vi "Analiza położeń robotów.vi"(0 "Zapis danych z przejazdu":T3={"Łazik"=path "C:/Users/User/Desktop/Łazik/Zapis zebranych danych/Łazik.txt", "Quadron"=path "C:/Users/User/Desktop/Łazik/Zapis zebranych danych/Łazik.txt", "Dron 1"=path "C:/Users/User/Desktop/Łazik/Zapis zebranych danych/Łazik.txt", "Dron 2"=path "C:/Users/User/Desktop/Łazik/Zapis zebranych danych/Łazik.txt", "Sparus"=path "C:/Users/User/Desktop/Łazik/Zapis zebranych danych/Łazik.txt"}, 1 "Azymut łazika\n pocz/nowy":dbl caption="Azymut robota pocz/nowy" min=0.0 max=360.0, 5 "Parametry odwzorowania\n Ziemi (WGS84)":T8={"a"=6378137.0, "b"=6356752.3142} {"b" format="%#.6g"; "a" format="%#.6g"}, 7 "Ustawienia początkowe":T5, 9 "Poł. bazy.":T7={"UTM"={"E [m]"=276177.7293177693, "N [m]"=1172675.379150019, "Strefa"="38P"}, "Piksele"={"X"=991, "Y"=338}} {"UTM"."N [m]" format="%#_10g"}, 11 "Wybór robota":T4 items=["Łazik", "Quadron", "Dron 1", "Dron 2"], 12 "Reset":T1) -> (4 "Azymut":dbl(knob) scale=0.0..360.0, 6 "Odległość robota od bazy  [m]":cluster{"X [m]":dbl, "Y [m]":dbl}, 10 "Lokalizacja robotów":T6, 15 "Odczyt GPS - Łazik 2":T2 caption="Położenie wybranego robota" {"Szerokośc geograficzna \n- GPS" format="%_9f"; "Długość geograficzna \n- GPS" format="%_9f"; "Położenie \nrobota  UTM"."E [m]" format="%#_10g"; "Położenie \nrobota  UTM"."N [m]" format="%#_12g"})   [LabVIEW 2015, in "Biblioteka moduł map v3.lvlib" / "Pomocnicze.lvlib"]
uses:
  Pomocnicze.lvlib
  Kontrolki/Parametry odwzorowania Ziemi.ctl
  Zmienne/Lokalizacja GPS/longitude Quadron.vi
  Zmienne/Lokalizacja GPS/latitude Quadron.vi
  Zmienne/Lokalizacja GPS/Longitude dron 1.vi
  Zmienne/Lokalizacja GPS/Latitude dron 1.vi
  Zmienne/Lokalizacja GPS/Latitude dron 2.vi
  Zmienne/Lokalizacja GPS/Longitude dron 2.vi
  Zmienne/Lokalizacja GPS/Longitude Sparus.vi
  Zmienne/Lokalizacja GPS/Latitude Sparus.vi
  Zmienne/Lokalizacja GPS/Lokalizacja GPS.lvlib
  Kontrolki/Kontrolki.lvlib
panel:
  # "Ta kkontrolka tylko dla łazika"
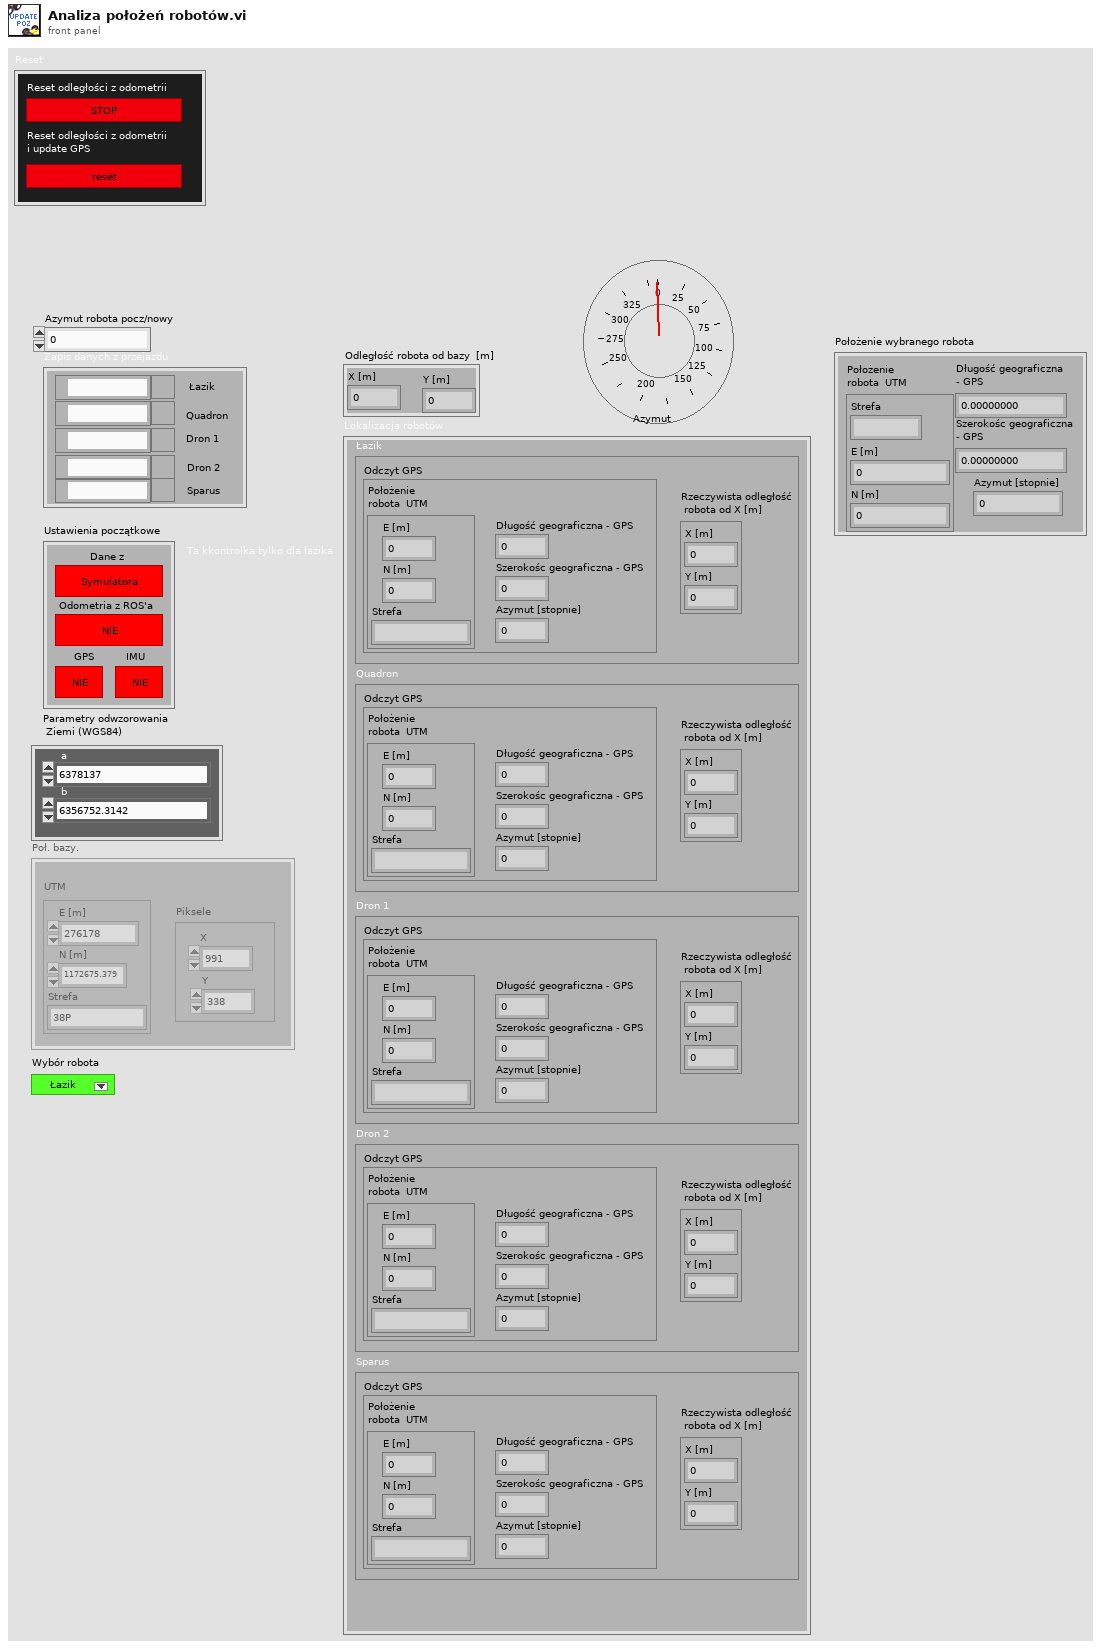
[diagram p1: front panel]
types:
  T1 = cluster{"reset odom":bool, "reset odom + gps":bool}
  T2 = cluster{"Położenie \nrobota  UTM":cluster{"E [m]":ext, "N [m]":ext, "Strefa":string}, "Długość geograficzna \n- GPS":dbl, "Szerokośc geograficzna \n- GPS":dbl, "Azymut [stopnie]":dbl}
  T3 = cluster{"Łazik":path, "Quadron":path, "Dron 1":path, "Dron 2":path, "Sparus":path}
  T4 = typedef "Biblioteka moduł map v3.lvlib/Kontrolki.lvlib/Wybór robota.ctl" = u16
  T5 = cluster{"Dane z":bool, "Odometria z ROS'a":bool, "GPS":bool, "IMU":bool}
  T6 = typedef "Biblioteka moduł map v3.lvlib/Kontrolki.lvlib/Lokalizacja robotów.ctl" = cluster{"Łazik":cluster{"Odczyt GPS":cluster{"Położenie \nrobota  UTM":cluster{"E [m]":ext, "N [m]":ext, "Strefa":string}, "Długość geograficzna - GPS":dbl, "Szerokośc geograficzna - GPS":dbl, "Azymut [stopnie]":dbl}, "Rzeczywista odległość\n robota od X [m]":cluster{"X [m]":dbl, "Y [m]":dbl}}, "Quadron":cluster{"Odczyt GPS":cluster{"Położenie \nrobota  UTM":cluster{"E [m]":ext, "N [m]":ext, "Strefa":string}, "Długość geograficzna - GPS":dbl, "Szerokośc geograficzna - GPS":dbl, "Azymut [stopnie]":dbl}, "Rzeczywista odległość\n robota od X [m]":cluster{"X [m]":dbl, "Y [m]":dbl}}, "Dron 1":cluster{"Odczyt GPS":cluster{"Położenie \nrobota  UTM":cluster{"E [m]":ext, "N [m]":ext, "Strefa":string}, "Długość geograficzna - GPS":dbl, "Szerokośc geograficzna - GPS":dbl, "Azymut [stopnie]":dbl}, "Rzeczywista odległość\n robota od X [m]":cluster{"X [m]":dbl, "Y [m]":dbl}}, "Dron 2":cluster{"Odczyt GPS":cluster{"Położenie \nrobota  UTM":cluster{"E [m]":ext, "N [m]":ext, "Strefa":string}, "Długość geograficzna - GPS":dbl, "Szerokośc geograficzna - GPS":dbl, "Azymut [stopnie]":dbl}, "Rzeczywista odległość\n robota od X [m]":cluster{"X [m]":dbl, "Y [m]":dbl}}, "Sparus":cluster{"Odczyt GPS":cluster{"Położenie \nrobota  UTM":cluster{"E [m]":ext, "N [m]":ext, "Strefa":string}, "Długość geograficzna - GPS":dbl, "Szerokośc geograficzna - GPS":dbl, "Azymut [stopnie]":dbl}, "Rzeczywista odległość\n robota od X [m]":cluster{"X [m]":dbl, "Y [m]":dbl}}}
  T7 = typedef "Biblioteka moduł map v3.lvlib/Kontrolki.lvlib/Położenie punktu bazowego.ctl" = cluster{"UTM":cluster{"E [m]":dbl, "N [m]":dbl, "Strefa":string}, "Piksele":cluster{"X":i32, "Y":i32}}
  T8 = typedef "Biblioteka moduł map v3.lvlib/Kontrolki.lvlib/Parametry odwzorowania Ziemi.ctl" = cluster{"a":dbl, "b":dbl}
  T9 = cluster{"Położenie \nrobota  UTM":cluster{"E [m]":ext, "N [m]":ext, "Strefa":string}, "Długość geograficzna - GPS":dbl, "Szerokośc geograficzna - GPS":dbl, "Azymut [stopnie]":dbl}
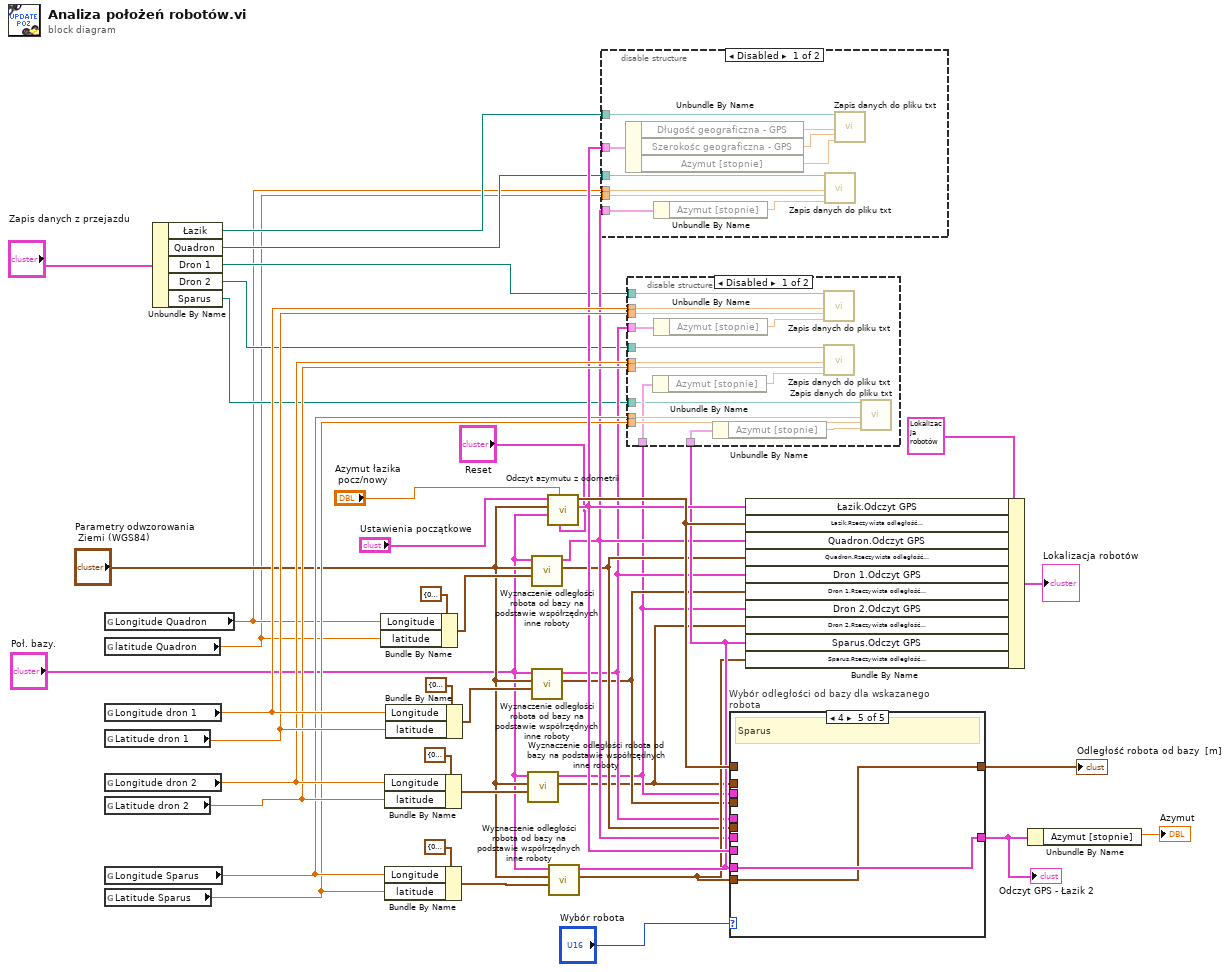
[diagram p0: block diagram]
diagram:
  n1 = global read "longitude Quadron.vi" "Longitude Quadron"() -> (w3:dbl)
  n2 = global read "latitude Quadron.vi" "latitude Quadron"() -> (w2:dbl)
  n3 = global read "Longitude dron 1.vi" "Longitude dron 1"() -> (w32:dbl)
  n4 = global read "Latitude dron 1.vi" "Latitude dron 1"() -> (w31:dbl)
  n5 = global read "Longitude dron 2.vi" "Longitude dron 2"() -> (w30:dbl)
  n6 = global read "Latitude dron 2.vi" "Latitude dron 2"() -> (w29:dbl)
  n7 = global read "Longitude Sparus.vi" "Longitude Sparus"() -> (w21:dbl)
  n8 = global read "Latitude Sparus.vi" "Latitude Sparus"() -> (w20:dbl)
  n9 = Unbundle By Name("Zapis danych z przejazdu") -> ("Łazik"=w8:path, "Quadron"=w7:path, "Dron 1"=w6:path, "Dron 2"=w5:path, "Sparus"=w4:path)
  n10 = Bundle By Name(cluster=cluster{"Longitude":dbl, "latitude":dbl} {"Longitude"=0.0, "latitude"=0.0} ("Lokalizacja robota GPS"), "Longitude"=w3, "latitude"=w2) -> (w40:cluster{"Longitude":dbl, "latitude":dbl})
  n11 = Bundle By Name(cluster=cluster{"Longitude":dbl, "latitude":dbl} {"Longitude"=0.0, "latitude"=0.0} ("Lokalizacja robota GPS"), "Longitude"=w30, "latitude"=w29) -> (w36:cluster{"Longitude":dbl, "latitude":dbl})
  n12 = Bundle By Name(cluster=cluster{"Longitude":dbl, "latitude":dbl} {"Longitude"=0.0, "latitude"=0.0} ("Lokalizacja robota GPS"), "Longitude"=w21, "latitude"=w20) -> (w23:cluster{"Longitude":dbl, "latitude":dbl})
  n13 = Bundle By Name(cluster=cluster{"Longitude":dbl, "latitude":dbl} {"Longitude"=0.0, "latitude"=0.0} ("Lokalizacja robota GPS"), "Longitude"=w32, "latitude"=w31) -> (w37:cluster{"Longitude":dbl, "latitude":dbl})
  n14 = call "Wyznaczenie odległości robota od bazy na podstawie współrzędnych inne roboty.vi"("Lokalizacja robota GPS"=w36, "Parametry odwzorowania Ziemi (WGS84)"="Parametry odwzorowania\n Ziemi (WGS84)", "Pocz. poł."="Poł. bazy.") -> ("Rzeczywista odległość robota od startu [m]"=w10:cluster{"X [m]":dbl, "Y [m]":dbl}, "Aktualne położenie"=w11:T9)  [unwired: 7 in]
  n15 = call "Wyznaczenie odległości robota od bazy na podstawie współrzędnych inne roboty.vi"("Lokalizacja robota GPS"=w40, "Parametry odwzorowania Ziemi (WGS84)"="Parametry odwzorowania\n Ziemi (WGS84)", "Pocz. poł."="Poł. bazy.") -> ("Rzeczywista odległość robota od startu [m]"=w14:cluster{"X [m]":dbl, "Y [m]":dbl}, "Aktualne położenie"=w15:T9)  [unwired: 7 in]
  n16 = call "Wyznaczenie odległości robota od bazy na podstawie współrzędnych inne roboty.vi"("Lokalizacja robota GPS"=w37, "Parametry odwzorowania Ziemi (WGS84)"="Parametry odwzorowania\n Ziemi (WGS84)", "Pocz. poł."="Poł. bazy.") -> ("Rzeczywista odległość robota od startu [m]"=w12:cluster{"X [m]":dbl, "Y [m]":dbl}, "Aktualne położenie"=w13:T9)  [unwired: 7 in]
  n17 = call "Odczyt azymutu z odometrii.vi"("Reset"="Reset", "Azymut robota\n pocz/nowy"="Azymut łazika\n pocz/nowy", "Położenie bazy"="Poł. bazy.", "Parametry odwzorowania Ziemi (WGS84)"="Parametry odwzorowania\n Ziemi (WGS84)", "Ustawienia początkowe"="Ustawienia początkowe") -> ("Odczyt GPS"=w28:T9, "Odległość robota od bazy [m]"=w34:cluster{"X [m]":dbl, "Y [m]":dbl})  [unwired: 4 in, 1 out]
  n18 = call "Wyznaczenie odległości robota od bazy na podstawie współrzędnych inne roboty.vi"("Lokalizacja robota GPS"=w23, "Parametry odwzorowania Ziemi (WGS84)"="Parametry odwzorowania\n Ziemi (WGS84)", "Pocz. poł."="Poł. bazy.") -> ("Rzeczywista odległość robota od startu [m]"=w16:cluster{"X [m]":dbl, "Y [m]":dbl}, "Aktualne położenie"=w17:T9)  [unwired: 7 in]
  n19 = disable-structure shown="Disabled" {
    disable-tunnel: w3 -> [w53 _]
    disable-tunnel: w2 -> [w52 _]
    disable-tunnel: w28 -> [w51 _]
    disable-tunnel: w15 -> [w50 _]
    disable-tunnel: w8 -> [w49 _]
    disable-tunnel: w7 -> [w48 _]
    frame Disabled {
      n20 = Unbundle By Name(w51) -> ("Długość geograficzna - GPS"=w47:dbl, "Szerokośc geograficzna - GPS"=w46:dbl, "Azymut [stopnie]"=w45:dbl)
      n21 = Unbundle By Name(w50) -> ("Azymut [stopnie]"=w44:dbl)
      n22 = call "Zapis danych do pliku txt.vi"("Dane zapisane z przejazdu \n(współrzędne, prędkości, azymut)"=w48, "Długość geograficzna - GPS"=w53, "Szerokośc geograficzna - GPS"=w52, "Azymut [stopnie]"=w44) -> ()  [unwired: 16 in]
      n23 = call "Zapis danych do pliku txt.vi"("Dane zapisane z przejazdu \n(współrzędne, prędkości, azymut)"=w49, "Długość geograficzna - GPS"=w47, "Szerokośc geograficzna - GPS"=w46, "Azymut [stopnie]"=w45) -> ()  [unwired: 16 in]
    }
    frame Enabled {
    }
  }
  n24 = disable-structure shown="Disabled" {
    disable-tunnel: w32 -> [w68 _]
    disable-tunnel: w31 -> [w67 _]
    disable-tunnel: w30 -> [w66 _]
    disable-tunnel: w29 -> [w65 _]
    disable-tunnel: w21 -> [w64 _]
    disable-tunnel: w20 -> [w63 _]
    disable-tunnel: w17 -> [w62 _]
    disable-tunnel: w13 -> [w61 _]
    disable-tunnel: w11 -> [w60 _]
    disable-tunnel: w6 -> [w59 _]
    disable-tunnel: w5 -> [w58 _]
    disable-tunnel: w4 -> [w55 _]
    frame Disabled {
      n25 = Unbundle By Name(w60) -> ("Azymut [stopnie]"=w57:dbl)
      n26 = Unbundle By Name(w61) -> ("Azymut [stopnie]"=w56:dbl)
      n27 = Unbundle By Name(w62) -> ("Azymut [stopnie]"=w54:dbl)
      n28 = call "Zapis danych do pliku txt.vi"("Dane zapisane z przejazdu \n(współrzędne, prędkości, azymut)"=w59, "Długość geograficzna - GPS"=w68, "Szerokośc geograficzna - GPS"=w67, "Azymut [stopnie]"=w56) -> ()  [unwired: 16 in]
      n29 = call "Zapis danych do pliku txt.vi"("Dane zapisane z przejazdu \n(współrzędne, prędkości, azymut)"=w58, "Długość geograficzna - GPS"=w66, "Szerokośc geograficzna - GPS"=w65, "Azymut [stopnie]"=w57) -> ()  [unwired: 16 in]
      n30 = call "Zapis danych do pliku txt.vi"("Dane zapisane z przejazdu \n(współrzędne, prędkości, azymut)"=w55, "Długość geograficzna - GPS"=w64, "Szerokośc geograficzna - GPS"=w63, "Azymut [stopnie]"=w54) -> ()  [unwired: 16 in]
    }
    frame Enabled {
    }
  }
  n31 = case "Wybór odległości od bazy dla wskazanego robota" shown="4" "Wybór robota" {
    tunnel: w34 -> [w70 _ _ _ _]
    tunnel: [w70 w72 w74 w76 w77] -> w33
    tunnel: w14 -> [_ w72 _ _ _]
    tunnel: w12 -> [_ _ w74 _ _]
    tunnel: w10 -> [_ _ _ w76 _]
    tunnel: w28 -> [w69 _ _ _ _]
    tunnel: [w69 w71 w73 w75 w78] -> w25
    tunnel: w15 -> [_ w71 _ _ _]
    tunnel: w13 -> [_ _ w73 _ _]
    tunnel: w11 -> [_ _ _ w75 _]
    tunnel: w17 -> [_ _ _ _ w78]
    tunnel: w16 -> [_ _ _ _ w77]
    frame 0, Default {
      # "Łazik"
    }
    frame 1 {
      # "Quadron"
    }
    frame 2 {
      # "Dron 1"
    }
    frame 3 {
      # "Dron 2"
    }
    frame 4 {
      # "Sparus"
    }
  }
  "Odległość robota od bazy  [m]" <- w33
  "Odczyt GPS - Łazik 2" <- w25
  n32 = Bundle By Name(cluster=T6 {"Łazik"={"Odczyt GPS"={"Położenie \nrobota  UTM"={"E [m]"=0.0, "N [m]"=0.0, "Strefa"=""}, "Długość geograficzna - GPS"=0.0, "Szerokośc geograficzna - GPS"=0.0, "Azymut [stopnie]"=0.0}, "Rzeczywista odległość\n robota od X [m]"={"X [m]"=0.0, "Y [m]"=0.0}}, "Quadron"={"Odczyt GPS"={"Położenie \nrobota  UTM"={"E [m]"=0.0, "N [m]"=0.0, "Strefa"=""}, "Długość geograficzna - GPS"=0.0, "Szerokośc geograficzna - GPS"=0.0, "Azymut [stopnie]"=0.0}, "Rzeczywista odległość\n robota od X [m]"={"X [m]"=0.0, "Y [m]"=0.0}}, "Dron 1"={"Odczyt GPS"={"Położenie \nrobota  UTM"={"E [m]"=0.0, "N [m]"=0.0, "Strefa"=""}, "Długość geograficzna - GPS"=0.0, "Szerokośc geograficzna - GPS"=0.0, "Azymut [stopnie]"=0.0}, "Rzeczywista odległość\n robota od X [m]"={"X [m]"=0.0, "Y [m]"=0.0}}, "Dron 2"={"Odczyt GPS"={"Położenie \nrobota  UTM"={"E [m]"=0.0, "N [m]"=0.0, "Strefa"=""}, "Długość geograficzna - GPS"=0.0, "Szerokośc geograficzna - GPS"=0.0, "Azymut [stopnie]"=0.0}, "Rzeczywista odległość\n robota od X [m]"={"X [m]"=0.0, "Y [m]"=0.0}}, "Sparus"={"Odczyt GPS"={"Położenie \nrobota  UTM"={"E [m]"=0.0, "N [m]"=0.0, "Strefa"=""}, "Długość geograficzna - GPS"=0.0, "Szerokośc geograficzna - GPS"=0.0, "Azymut [stopnie]"=0.0}, "Rzeczywista odległość\n robota od X [m]"={"X [m]"=0.0, "Y [m]"=0.0}}} ("Lokalizacja robotów"), "Łazik.Odczyt GPS"=w28, "Łazik.Rzeczywista odległość\n robota od X [m]"=w34, "Quadron.Odczyt GPS"=w15, "Quadron.Rzeczywista odległość\n robota od X [m]"=w14, "Dron 1.Odczyt GPS"=w13, "Dron 1.Rzeczywista odległość\n robota od X [m]"=w12, "Dron 2.Odczyt GPS"=w11, "Dron 2.Rzeczywista odległość\n robota od X [m]"=w10, "Sparus.Odczyt GPS"=w17, "Sparus.Rzeczywista odległość\n robota od X [m]"=w16) -> (→"Lokalizacja robotów":T6)
  n33 = Unbundle By Name(w25) -> ("Azymut [stopnie]"=→"Azymut":dbl)
